vi "test.vi"() -> ()   [LabVIEW 2009]
panel:
  out "error type":enum16{"fatal", "non-fatal", "warning"}(ring)
  in  "VIs without test coverage":i32(listbox)
  out "error out":errorcluster
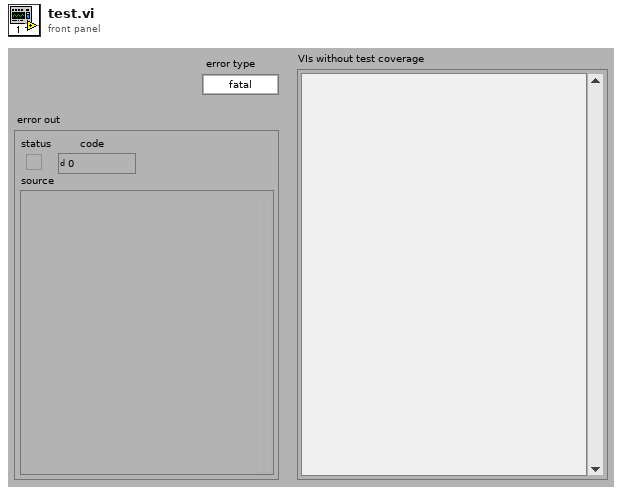
[diagram p1: front panel]
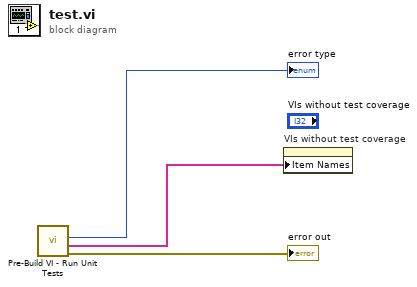
[diagram p0: block diagram]
diagram:
  n1 = call "Pre-Build VI - Run Unit Tests.vi"() -> ("error out"=→"error out":errorcluster, "VIs without test coverage"=w2:string[], "error type"=→"error type":enum16{"fatal", "non-fatal", "warning"})  [unwired: 9 in]
  n2 = property on="VIs without test coverage" class="ListBox (strict)"("Item Names"=w2) -> ()  [unwired: 2 in, 2 out]
